vi "Z Go.vi"(8 "error in (no error)":errorcluster, 9 "Speed":dbl format="%#_13g", 10 "Position":dbl format="%#_13g", 11 "Gantry 2":refnum<k24>) -> (0 "error out":errorcluster, 3 "Gantry 3":refnum<k24>)   [LabVIEW 2020, in "A3200.lvclass"]
uses:
  A3200.lvclass
  C:/Program Files (x86)/Aerotech/A3200/LabVIEW/2010/Bin/Aerotech.A3200.dll
  Program Files (x86)/Aerotech/A3200/LabVIEW/2010/Bin/Aerotech.A3200.dll
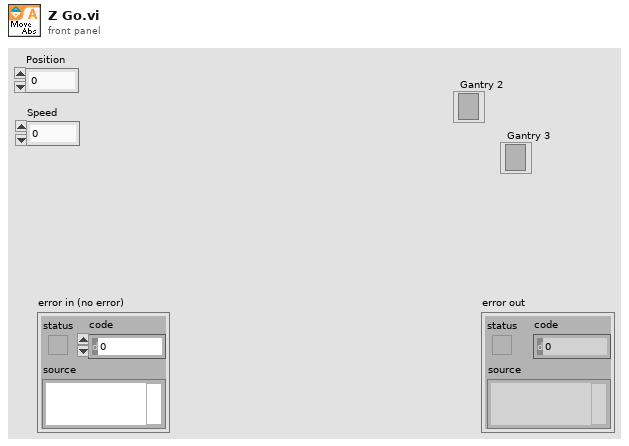
[diagram p1: front panel]
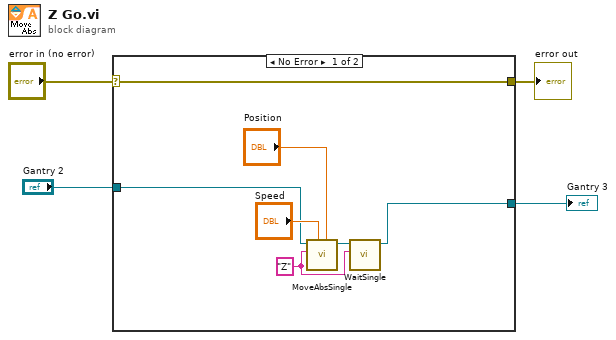
[diagram p0: block diagram]
diagram:
  n1 = case shown="No Error" "error in (no error)" {
    selector: "error in (no error)" -> [w11 w12]
    tunnel: [w11 w12] -> w3
    tunnel: "Gantry 2" -> [w6 _]
    tunnel: [w5 _] -> w1
    frame No Error {
      w7 = "Z"
      n2 = call "MoveAbsSingle.vi"("position"="Position", "speed"="Speed", "axis name"=w7, "controller in"=w6) -> ("controller out"=w10:refnum<k24>)  [unwired: 6 in, 1 out]
      n3 = call "WaitSingle.vi"("axis name"=w7, "controller in"=w10) -> ("controller out"=w5:refnum<k24>)  [unwired: 7 in, 2 out]
    }
    frame Error {
    }
  }
  "error out" <- w3
  "Gantry 3" <- w1
